vi "AlliGator Init Settings v2.vi"(8 "error in":errorcluster, 10 "Parameters to set to Default":T1[](array[typedef]), 11 "Settings Panel (Empty: All)":string) -> (0 "error out":errorcluster)   [LabVIEW 2021, in "AlliGator Settings.lvlib"]
doc: "Resets selected Settings parameters to their default values."
uses:
  AlliGator Settings.lvlib
  AlliGator Settings List.ctl
  Arrays/Linear Ramp End Options.ctl
  AlliGator Settings Event.ctl
  AlliGator Settings Window Messages.ctl
  AlliGator Define Gates to.ctl
  AlliGator Gates to Skip.ctl
  AlliGator Average Lifetime Options.ctl
  Fits/IRF(X)PSED/IRF(X)PSED Extraction Options.ctl
  Fits/IRF(X)PSED/Fourier Series Smoothing Option.ctl
  Fits/IRF(X)PSED/Fourier Series Truncation.ctl
  Fits/IRF(X)PSED/IRF Extraction Method.ctl
  AlliGator IRF Optimization Controls.ctl
  AlliGator IRF Deconvolution Metrics.ctl
  Fits/Square Pulse/Square Pulse Options.ctl
  Fits/Square Pulse/Square Pulse Levels Type.ctl
  Math/Advanced Signal Processing Toolkit/Wavelet Analysis Options.ctl
  AlliGator Baseline Subtraction Method.ctl
  Graphs/XY Graph/XY Graph Plot Shift Parameters.ctl
  Graphs/XY Graph/XY Graph Plot Shift Method.ctl
  Fits/IRF(X)PSED/Decay Fit Options v2.ctl
  Fits/Decay Convolution/Decay Model.ctl
  Fits/Residual Type.ctl
  Fits/IRF(X)PSED/Fit Weights Type.ctl
  Fits/Non-linear Fitting Method v2.ctl
  Fits/Fit Calculation Method.ctl
  Fits/Non-linear Fitting Algorithm.ctl
  Fits/IRF(X)PSED/Decay Fit Parameters & Derived Quantities List.ctl
  AlliGator Decay Fit Parameter Constraints 2.ctl
  Fits/IRF(X)PSED/Decay Fit Parameters In List.ctl
  AlliGator Guess Parameters Options.ctl
  Fits/IRF(X)PSED/MLE Baseline Offset Type.ctl
  AlliGator Exported Image Settings.ctl
  Histograms/Linear Histogram Options.ctl
  Histograms/Histogram Bin Option.ctl
  Histograms/Histogram Bin Position.ctl
  Image/Image Save File Format.ctl
  AlliGator Calibration Map Algorithm.ctl
  Phasor/Phasor Calibration Type.ctl
  AlliGator Phasor Reference Associated with Shortest Lifetime.ctl
  Phasor/Phasor Ratio Type.ctl
  Phasor/Phasor Standard Deviation Options.ctl
  AlliGator Phasor Plot Graphics Options.ctl
  AlliGator Phasor Plot Size.ctl
  AlliGator Phasor Plot Smoothing Options.ctl
  Arrays/Kernel Type.ctl
  Arrays/Smoothing Algorithm.ctl
  AlliGator Phasor Ratio Color-Coded Quantity.ctl
  AlliGator Python Settings.ctl
  Phasor/Phasor Explorer Decay Parameters.ctl
  Phasor/Phasor IRF Model.ctl
  Phasor/Phasor Explorer Display Parameters.ctl
  Phasor/Phasor Type of Series.ctl
  Phasor/Phasor Explorer Gate Parameters.ctl
  Phasor/Phasor Gate Type.ctl
  Phasor/Phasor Type of User-defined Function.ctl
  Phasor/Phasor Explorer Phasor Parameters.ctl
  Phasor/Phasor Calculation Type.ctl
  Phasor/Phasor SEPL Type.ctl
  Graphs/XY Graph/XY Plot Data.ctl
  AlliGator High Count Pixels Rejection Options.ctl
  SwissSPAD/SwissSPAD Live_Image Display Options.ctl
  AlliGator Image Binning Options.ctl
  AlliGator Image Smoothing Options.ctl
  AlliGator Low Count Pixels Rejection Options.ctl
  AlliGator Source Image Scale Bar Options.ctl
  Image/Flatfield Correction Options.ctl
  528bb3ad-a7d6-4b51-8aeb-33b87c87e59f.vi
  7656f502-c6d9-4b62-8342-3e3474e45c54.vi
  7a1d85e8-f51a-467b-92ae-4795812e884b.vi
  48533959-b6d0-4ae5-a5e9-0e715072b6cc.vi
  d87100d8-5b63-464b-a767-9d3b270a4e3f.vi
  7656f502-c6d9-4b62-8342-3e3474e45c54.vi/539bd7ec-d9e8-460f-a56d-a449b4a86a5e.vi
  7a1d85e8-f51a-467b-92ae-4795812e884b.vi/539bd7ec-d9e8-460f-a56d-a449b4a86a5e.vi
  48533959-b6d0-4ae5-a5e9-0e715072b6cc.vi/539bd7ec-d9e8-460f-a56d-a449b4a86a5e.vi
  d87100d8-5b63-464b-a767-9d3b270a4e3f.vi/539bd7ec-d9e8-460f-a56d-a449b4a86a5e.vi
  AlliGator Decay Analysis.lvlib
  Graphs/XY Graph/XY Graph Add-Ons.lvlib
  AlliGator Phasor Plot.lvlib
  Image/Image.lvlib
  AlliGator Decay Preprocessing.lvlib
  Fits/Fits.lvlib
  AlliGator Decay Fit.lvlib
  AlliGator IRF.lvlib
  Math/Math.lvlib
  Arrays/Arrays.lvlib
  Strings/Strings.lvlib
  AlliGator Source Image.lvlib
  Phasor/Phasor Explorer.lvlib
  Phasor/Phasor.lvlib
  AlliGator Phasor Ratio.lvlib
  Histograms/Histogram Window.lvlib
  AlliGator Phasor Calibration.lvlib
  SwissSPAD/SwissSPAD Live.lvlib
panel:
  # "see the AlliGator License on the block diagram (Ctrl+E or Window:Show Block Diagram)"
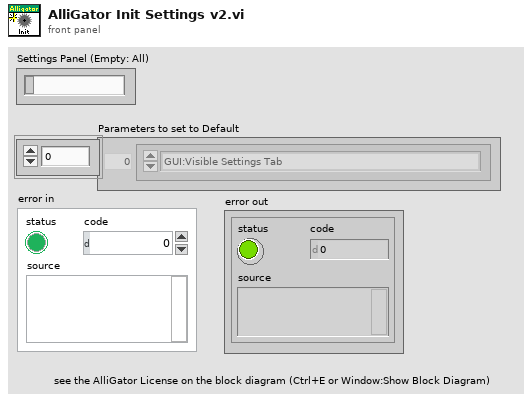
[diagram p1: front panel]
types:
  T1 = typedef "AlliGator Settings.lvlib/AlliGator Settings List.ctl" = enum16{"GUI:Visible Settings Tab", "GUI:Last Run Version", "Source Image:Use Image Histogram for Contrast", "Source Image:Low Count Pixels Rejection Options", "Source Image:High Count Pixels Rejection Options", "Source Image:Use Image Brightness", "Source Image:Blend Overlay with Image Background", "Source Image:Use Fixed ROI Diameter", "Source Image:ROI Diameter", "Source Image:ROI Center Color", "Source Image:Peak Threshold", "Source Image:Intensity Threshold", "Source Image:Image Binning Options", "Source Image:Image Smoothing Options", "Source Image:Image Histogram Active", "Source Image:Invert Binary Mask", "Source Image:Hot Pixel Removal", "Source Image:Overlay Analyzed ROI Center", "Source Image:Auto-Adjust Contrast", "Source Image:Histogram Lower Percentile", "Source Image:Histogram Upper Percentile", "Source Image:Save Source Image", "Source Image:Scale Bar Options", "Source Image:Image Resolution (Pixel Size)", "Source Image:Flatfield Correction", "Source Image:Show Dead Left Columns Correction", "Source Image:Dead Left Columns Correction", "Source Image:Image Pre-Processing Operations Order", "Source Image:Overlay ROI Median", "Source Image:Median Overlay Color", "Data Information:Gate Width", "Data Information:Nanotime Gate Separation", "Data Information:Macrotime Gate Separation", "Data Information:Gate Step", "Data Information:# Gates", "Data Information:Gate Image Exposure", "Data Information:Gate Image Integration", "Data Information:Gates to Skip", "Data Information:Gates to Keep", "Data Information:Define Gates to", "Data Information:Channel Name", "Data Information:Available Channel Names", "Data Information:Channel Arithmetic", "Data Information:Background File Subtraction", "Data Information:Background File", "Data Information:Background Scaling Factor", "Data Information:Background Pile-up Correction", "Data Information:Background Pixel Well Capacity", "Data Information:Laser Period", "Data Information:SYNC Period", "Data Information:Pile-up Correction", "Data Information:Pixel Well Capacity", "Data Information:Dataset Scaling Factor", "Fluorescence Decay_Decay Pre-Processing:Reverse Gates", "Fluorescence Decay_Decay Pre-Processing:Verbose Decay Pre-Processing", "Fluorescence Decay_Decay Pre-Processing:Use Decay Pre-Processing", "Fluorescence Decay_Decay Pre-Processing:Background Subtraction", "Fluorescence Decay_Decay Pre-Processing:Background Definition Range", "Fluorescence Decay_Decay Pre-Processing:Baseline Subtraction Method", "Fluorescence Decay_Decay Pre-Processing:Decay Pre-Processing Operations Order", "Fluorescence Decay_Decay Pre-Processing:Smoothing Parameter", "Fluorescence Decay_Decay Pre-Processing:Shift Decay", "Fluorescence Decay_Decay Pre-Processing:Decay Shift Parameters", "Fluorescence Decay_Decay Pre-Processing:Fold Decay", "Fluorescence Decay_Decay Pre-Processing:# Folds", "Fluorescence Decay_Decay Pre-Processing:1-Normalize Decay", "Fluorescence Decay_Decay Pre-Processing:[0-1]-Normalize Decay", "Fluorescence Decay_Decay Pre-Processing:Smoothen Decay", "Fluorescence Decay_Decay Pre-Processing:Extrapolate Decay", "Fluorescence Decay_Decay Pre-Processing:Use Periodicity", "Fluorescence Decay_Decay Pre-Processing:Use Cursors", "Fluorescence Decay_Decay Pre-Processing:Tail Fraction", "Fluorescence Decay_Decay Pre-Processing:Head Fraction", "Fluorescence Decay_Decay Pre-Processing:Additional Points", "Fluorescence Decay_Decay Pre-Processing:Straighten Decay", "Fluorescence Decay_Decay Pre-Processing:Constant Background", "Fluorescence Decay_Decay Pre-Processing:Pixel-Normalize Decay", "Fluorescence Decay_Advanced Analysis:Extract IRF instead of Decay", "Fluorescence Decay_Advanced Analysis:IRF Extraction Options", "Fluorescence Decay_Advanced Analysis:IRF Optimization Options", "Fluorescence Decay_Advanced Analysis:Square Pulse Options", "Fluorescence Decay_Advanced Analysis:IRF Order", "Fluorescence Decay_Advanced Analysis:IRF Time Constants", "Fluorescence Decay_Advanced Analysis:Wavelet Analysis Options", "Fluorescence Decay_Advanced Analysis:Average Lifetime Options", "Fluorescence Decay_Fit Options:Fit Options", "Fluorescence Decay_Fit Options:Use Legacy Fitting Approach", "Fluorescence Decay_Fit Options:Use Data Information Laser Period", "Fluorescence Decay_Fit Parameters:Displayed Fit Parameters", "Fluorescence Decay_Fit Parameters:Fit Parameter Constraints", "Fluorescence Decay_Fit Parameters:Export Tabulated Results", "Fluorescence Decay_Fit Parameters:MLE Baseline Offset Type", "Fluorescence Decay_Fit Parameters:MLE Baseline Offset", "Fluorescence Decay_Fit Parameters:Guess Parameter Names", "Fluorescence Decay_Fit Parameters:Guess Parameter Values", "Fluorescence Decay_Fit Parameters:Guess Parameters Options", "Fluorescence Decay_Styles:Show Last Decay Only", "Fluorescence Decay_Styles:Decay Graph Color Array", "Fluorescence Decay:Decay Graph Active", "Fluorescence Decay Statistics:Min Peak Value", "Fluorescence Decay Statistics:Reject Low Decay Peak Pixels", "Fluorescence Decay Statistics:Reject High Decay Peak Pixels", "Fluorescence Decay Statistics:Max Peak Value", "Time Traces:Use File Timestamp", "Time Traces:Time Step", "Time Traces:Use Intensity Correction File", "Time Traces:Intensity Correction File", "Phasor Plot:Phasor Plot Smoothing Options", "Phasor Plot:Phasor Plot Size", "Phasor Plot:Phasor Plot Graphics Options", "Phasor Plot:Cumulative Phasor Plot", "Phasor Plot:Use Phasor Brightness", "Phasor Plot:Blend Overlay with Phasor Background", "Phasor Plot:Save Phasor Plot", "Phasor Plot:Show References", "Phasor Plot:Phasor Ratio Decay Range", "Phasor Plot:Exponential Fading", "Phasor Plot:Phasor Ratio Reference Colors", "Phasor Plot:Reference Radius", "Phasor Plot:Show Color Map Vertices", "Phasor Plot:Phasor Plot Active", "Phasor Plot:Phasor Ratio Color Map Type", "Phasor Plot:Phasor Ratio Color Map", "Phasor Plot:Phasor Ratio Display Range", "Phasor Plot:Selected Image ROI(s)", "Phasor Plot:All Image ROIs", "Phasor Plot:Selected Phasor Plot ROI(s)", "Phasor Plot:All Phasor Plot ROIs", "Phasor Plot:Phasor Ratio Color-Coded Quantity", "Phasor Plot:Store Phasor Harmonics", "Phasor Plot:Draw Reference Segment", "Phasor Plot:User-Defined Quantity", "Phasor Graph:Phasor Frequency", "Phasor Graph:Phasor Ratio Type", "Phasor Graph:Pixel-level Phasor Computation", "Phasor Graph:Save Phasor Graph", "Phasor Graph:Phasor Graph Active", "Phasor Graph:Phasor SDV Options", "Phasor Calibration:Use Backup Calibration if needed", "Phasor Graph:Define Shortest Lifetime as", "Phasor Calibration:Backup Calibration Type", "Phasor Calibration:Calibration Type", "Phasor Calibration:Calibration Lifetime", "Phasor Calibration:Calibration Map Algorithm", "Single-Exponential Phasor Locus (SEPL):Gate Parameters", "Single-Exponential Phasor Locus (SEPL):User-defined Gate", "Single-Exponential Phasor Locus (SEPL):User-defined IRF", "Single-Exponential Phasor Locus (SEPL):Phasor Parameters", "Single-Exponential Phasor Locus (SEPL):Decay & IRF Parameters", "Single-Exponential Phasor Locus (SEPL):Display Parameters", "Lifetime Analysis:Decay Analysis Parameters", "Lifetime Analysis:Lifetime Map Active", "Plugins:Python Settings", "Miscellaneous:Verbose Mode", "Miscellaneous:Beep after Script", "Miscellaneous:Saved Image File Format", "Miscellaneous:Exported Gate Image Settings", "Miscellaneous:Include Loading in Timing", "Miscellaneous:Verbose Settings Mode", "Miscellaneous:Histogram Options", "Miscellaneous:Beep on Error", "Miscellaneous:# Logical Processors Used", "Miscellaneous:ROI Description Max Characters", "Miscellaneous:Verbose Error Mode", "Miscellaneous:Transparent Mask Color"}
  T2 = typedef "Arrays.lvlib/Linear Ramp End Options.ctl" = enum16{"Include Min/Exclude Max", "Exclude Min/Include Max", "Include Both Ends", "Exclude Both Ends"}
  T3 = typedef "AlliGator Settings.lvlib/AlliGator Settings Event.ctl" = cluster{"AlliGator Settings Message":T4, "Sender":string, "Control Label":string, "Data":variant}
  T4 = typedef "AlliGator Settings.lvlib/AlliGator Settings Window Messages.ctl" = enum16{"Idle", "Subscribe", "Unsubscribe", "Refresh Parameter", "Refresh All Parameters", "Quit"}
  T5 = typedef "AlliGator Settings.lvlib/AlliGator Define Gates to.ctl" = enum32{"Skip", "Keep"}
  T6 = typedef "AlliGator Decay Analysis.lvlib/AlliGator Gates to Skip.ctl" = cluster{"Start":u32, "End":u32}
  T7 = typedef "AlliGator Settings.lvlib/AlliGator Average Lifetime Options.ctl" = cluster{"Use Local IRF ":bool, "Use IRF Offset":bool, "Use Fixed Offset":bool, "Fixed Offset":dbl[unit], "Baseline %":dbl}
  T8 = typedef "Fits.lvlib/IRF(X)PSED Extraction Options.ctl" = cluster{"Time Constant for IRF Extraction":dbl[unit], "IRF Order":i32, "Fourier Series Smoothing":T9, "Noise Threshold":dbl, "Smoothing Width":dbl, "Fourier Series Truncation":T10, "Truncation Order":i32, "Save Power Spectrum":bool, "Smoothing":bool, "Smoothing Parameter":dbl, "Smoothing Order":u32, "Method":T11}
  T9 = typedef "Fits.lvlib/Fourier Series Smoothing Option.ctl" = enum16{"None", "Lanczos Factors", "Fejer Summation"}
  T10 = typedef "Fits.lvlib/Fourier Series Truncation.ctl" = enum16{"Automatic", "Fixed"}
  T11 = typedef "Fits.lvlib/IRF Extraction Method.ctl" = enum16{"Direct", "Topless", "Toeplitz"}
  T12 = typedef "AlliGator Decay Analysis.lvlib/AlliGator IRF.lvlib/AlliGator IRF Optimization Controls.ctl" = cluster{"Search Range":dbl[unit], "Search Step":dbl[unit], "Tail Threshold (%)":dbl, "Regularized IRF":bool, "Export Plot":bool, "Export Data":bool, "Smooth Metrics":bool, "S-G Side Points":i32, "S-G Polynomial Order":i32, "Metrics":T13}
  T13 = typedef "AlliGator Decay Analysis.lvlib/AlliGator IRF.lvlib/AlliGator IRF Deconvolution Metrics.ctl" = enum16{"Average", "SDV", "Max", "Average * SDV", "Slope"}
  T14 = typedef "Fits.lvlib/Square Pulse Options.ctl" = cluster{"Method":T15, "# Bins":i32, "Threshold %":dbl, "Center on Midpoint":bool, "Smoothen Plot":bool}
  T15 = typedef "Fits.lvlib/Square Pulse Levels Type.ctl" = enum16{"Mode", "Mean"}
  T16 = typedef "Math.lvlib/Wavelet Analysis Options.ctl" = cluster{"Wavelet":enum16{"db02", "db03", "db04", "db05", "db06", "db07", "db08", "db09", "db10", "db11", "db12", "db13", "db14", "Haar", "bior1_3", "bior1_5", "bior2_2", "bior2_4", "bior2_6", "bior2_8", "bior3_1", "bior3_3", "bior3_5", "bior3_7", "bior3_9", "bior4_4 (FBI)", "bior5_5", "bior6_8", "coif1", "coif2", "coif3", "coif4", "coif5", "sym2", "sym3", "sym4", "sym5", "sym6", "sym7", "sym8"}, "Option for Approximate Coefficients":enum16{"None", "Threshold", "Detrend"}, "# Levels":i32, "Threshold Settings":cluster{"Thresholding Rule":enum16{"SURE", "Hybrid", "Universal", "Minimax"}, "Rescaling Method":enum16{"One", "Single level", "Multiple levels"}, "Soft Threshold?":bool}, "Wavelet Transform Type":enum16{"Discrete", "Undecimated"}}
  T17 = cluster{"Min Gate":dbl[unit], "Max Gate":dbl[unit]}
  T18 = typedef "AlliGator Decay Analysis.lvlib/AlliGator Decay Preprocessing.lvlib/AlliGator Baseline Subtraction Method.ctl" = enum16{"Mean", "Min", "Square Gated Single-Exponential", "File", "Constant"}
  T19 = typedef "XY Graph Add-Ons.lvlib/XY Graph Plot Shift Parameters.ctl" = cluster{"Type":T20, "Shift":dbl[unit], "Threshold":dbl, "Rotate":bool}
  T20 = typedef "XY Graph Add-Ons.lvlib/XY Graph Plot Shift Method.ctl" = enum16{"Default", "CFD", "Threshold", "Cross-Correlation"}
  T21 = typedef "Fits.lvlib/Decay Fit Options v2.ctl" = cluster{"Show Fit Residuals":bool, "Fit Model":T22, "Residual Type":T23, "Max Decay Percentile":dbl, "Min Decay Percentile":dbl, "Show Full Decay":bool, "Weights":T24, "Fitting Method":T25, "Compute Parameter Uncertainties":bool, "Periodic Boundaries":bool, "Model Calculation":T26, "Period":dbl[unit], "Termination Criteria":cluster{"Max Iterations":i32, "Max Function Calls":i32, "Max Time":dbl[unit], "Function Tolerance":dbl, "Parameter Tolerance":dbl, "Gradient Tolerance":dbl, "Min Lambda":dbl, "Max Lambda":dbl, "Initial Tick Count":u32}, "Offset Resolution":dbl[unit], "Use Local IRF":bool, "Fitting Algorithm":T27}
  T22 = typedef "Fits.lvlib/Decay Model.ctl" = enum16{"1-Exponential", "2-Exponentials"}
  T23 = typedef "Fits.lvlib/Residual Type.ctl" = enum16{"Standard", "Normalized", "Reduced"}
  T24 = typedef "Fits.lvlib/Fit Weights Type.ctl" = enum16{"Unweighted", "1/Variance", "Best of All"}
  T25 = typedef "Fits.lvlib/Non-linear Fitting Method v2.ctl" = enum16{"Least Square", "Least Absolute Residual", "Bisquare", "MLE", "-", "Best of All"}
  T26 = typedef "Fits.lvlib/Fit Calculation Method.ctl" = enum16{"Simulation", "Convolution", "Integration"}
  T27 = typedef "Fits.lvlib/Non-linear Fitting Algorithm.ctl" = enum16{"Levenberg-Marquardt", "Trust-Region Dogleg"}
  T28 = typedef "AlliGator Decay Analysis.lvlib/AlliGator Decay Fit.lvlib/AlliGator Decay Fit Parameter Constraints 2.ctl" = cluster{"Fit Parameter":T29, "Min Value":dbl, "Max Value":dbl, "Global":bool, "Used":bool}
  T29 = typedef "Fits.lvlib/Decay Fit Parameters In List.ctl" = enum16{"Offset", "Baseline", "A_1", "tau_1", "A_2", "tau_2"}
  T30 = typedef "AlliGator Decay Analysis.lvlib/AlliGator Decay Fit.lvlib/AlliGator Guess Parameters Options.ctl" = enum16{"Numerically estimated", "User-provided", "User-provided (normalized)", "Last valid fitted parameters"}
  T31 = typedef "Fits.lvlib/MLE Baseline Offset Type.ctl" = enum32{"Absolute", "Percentage"}
  T32 = typedef "AlliGator Settings.lvlib/AlliGator Exported Image Settings.ctl" = cluster{"bitness":bool, " Min Value":sgl, " Max Value":sgl}
  T33 = typedef "Histogram Window.lvlib/Linear Histogram Options.ctl" = cluster{"Bin Size":dbl, "Bin Number":i32, "Bin Option":T34, "Min Value":dbl, "Max Value":dbl, "Filter NaN & Infinite Values":bool, "Frequency Plot":bool, "Align Bins":bool, "Bin Location":T35, "Project Outside Values":bool, "Max Histogram Size":i32}
  T34 = typedef "Histogram Window.lvlib/Histogram Bin Option.ctl" = enum32{"Bin Number", "Bin Size"}
  T35 = typedef "Histogram Window.lvlib/Histogram Bin Position.ctl" = enum16{"Left", "Center", "Right"}
  T36 = typedef "Image.lvlib/Image Save File Format.ctl" = enum16{"PNG", "JPEG", "BMP"}
  T37 = enum16{"Single Calibration", "Nearest Valid Calibration"}
  T38 = typedef "AlliGator Phasor Calibration.lvlib/AlliGator Calibration Map Algorithm.ctl" = enum16{"Simple Search", "Min Distance"}
  T39 = typedef "Phasor.lvlib/Phasor Calibration Type.ctl" = enum16{"None", "Single Phasor", "Phasor Series", "Phasor Map"}
  T40 = typedef "AlliGator Phasor Ratio.lvlib/AlliGator Phasor Reference Associated with Shortest Lifetime.ctl" = enum32{"Reference 1", "Reference 2"}
  T41 = typedef "Phasor.lvlib/Phasor Ratio Type.ctl" = enum32{"Intensity-weighted", "Amplitude-weighted"}
  T42 = typedef "Phasor.lvlib/Phasor Standard Deviation Options.ctl" = cluster{"Compute Estimated SDV":bool, "# Replicas":u32, "Use Estimated Average Phasor":bool}
  T43 = typedef "AlliGator Settings.lvlib/AlliGator Phasor Plot Graphics Options.ctl" = cluster{"UC Color":u32, "Show UC Tau Ticks":bool, "SEPL Color":u32, "Show SEPL Tau Ticks":bool, "Axes Color":u32, "Show (g,s) Ticks":bool, "Show UC":bool, "Show SEPL":bool, "Show Axes":bool, "Show UC Tau Labels":bool, "Show SEPL Tau Labels":bool, "Show (g,s) Labels":bool, "UC Label Size":i16, "UC Label Distance":dbl, "SEPL Label Size":i16, "SEPL Label Distance":dbl, "Axes Label Size":i16, "Axes Label Distance":dbl}
  T44 = typedef "AlliGator Phasor Plot.lvlib/AlliGator Phasor Plot Size.ctl" = cluster{"H":i32, "V":i32, "Margin":dbl}
  T45 = typedef "AlliGator Phasor Plot.lvlib/AlliGator Phasor Plot Smoothing Options.ctl" = cluster{"Use Phasor Plot Smoothing":bool, "Kernel Type":T46, "Bin":i32, "Algorithm":T47}
  T46 = typedef "Arrays.lvlib/Kernel Type.ctl" = enum16{"Uniform", "Bilinear", "Gaussian"}
  T47 = typedef "Arrays.lvlib/Smoothing Algorithm.ctl" = enum16{"Rapid", "Thorough"}
  T48 = enum32{"Interpolate Reference Colors", "Use Custom Map"}
  T49 = typedef "AlliGator Phasor Ratio.lvlib/AlliGator Phasor Ratio Color-Coded Quantity.ctl" = enum16{"Phasor Ratio (f1 or a1)", "Average Lifetime (<tau>_i or <tau>_a))", "User-Defined Quantity"}
  T50 = cluster{"Reference 1":u32, "Reference 2":u32, "Boundary":u32}
  T51 = typedef "AlliGator Settings.lvlib/AlliGator Python Settings.ctl" = cluster{"Python Version":string, "Use PATH definition":bool, "Python.exe Path":path, "Include Example Plugins":bool}
  T52 = typedef "Phasor Explorer.lvlib/Phasor Explorer Decay Parameters.ctl" = cluster{"Lifetime":dbl[unit], "IRF Offset":dbl[unit], "IRF Period":dbl[unit], "Normalized Decays":bool, "IRF Model":T53, "IRF Parameter 1":dbl[unit]}
  T53 = typedef "Phasor.lvlib/Phasor IRF Model.ctl" = enum16{"Dirac", "Exponential"}
  T54 = typedef "Phasor Explorer.lvlib/Phasor Explorer Display Parameters.ctl" = cluster{"# Points":i32, "Ramp Type":enum16{"Linear", "Logarithmic"}, "Type of Series":T55, "Min tau":dbl[unit], "Max tau":dbl[unit], "Include 0":bool, "Include Infinity":bool}
  T55 = typedef "Phasor.lvlib/Phasor Type of Series.ctl" = enum16{"1-Exp Decays", "Linear Combination of 1-Exp"}
  T56 = typedef "Phasor Explorer.lvlib/Phasor Explorer Gate Parameters.ctl" = cluster{"First Gate Start":dbl[unit], "Use Gate Center":bool, "Gate Width":dbl[unit], "Gate Step":dbl[unit], "# Gates":dbl, "Gate Type":T57, "Edge Width":dbl[unit], "Top Slope":dbl[unit], "Reversed Sawtooth?":bool, "Analytical Computation":bool, "Integration":enum32{"Item 0", "Item 1"}, "Tolerance":dbl, "# Steps":dbl, "Type of User-defined Function":T58, "Use Gate Step":bool}
  T57 = typedef "Phasor.lvlib/Phasor Gate Type.ctl" = enum16{"Square", "Finite Edge Square", "Finite Edge, Tilted Top Square", "Triangle", "Sawtooth", "User-defined"}
  T58 = typedef "Phasor.lvlib/Phasor Type of User-defined Function.ctl" = enum16{"Gate", "IRF"}
  T59 = typedef "Phasor Explorer.lvlib/Phasor Explorer Phasor Parameters.ctl" = cluster{"Harmonic Frequency":dbl[unit], "Use f* = 1/D Frequency":bool, "Calibrated Phasor":bool, "Calibration Lifetime":dbl[unit], "Phasor Calculation":T60, "SEPL Type":T61, "# Gates":dbl, "Square Gate Width":dbl[unit], "Show Ticks":bool}
  T60 = typedef "Phasor.lvlib/Phasor Calculation Type.ctl" = enum16{"Direct Sum", "Analytical Formula"}
  T61 = typedef "Phasor.lvlib/Phasor SEPL Type.ctl" = enum16{"UC", "L_N", "L_N[W]", "L_X"}
  T62 = typedef "XY Graph Add-Ons.lvlib/XY Plot Data.ctl" = cluster{"X Array":dbl[], "Y Array":dbl[]}
  T63 = typedef "AlliGator Settings.lvlib/AlliGator High Count Pixels Rejection Options.ctl" = cluster{"Background High Threshold Factor":dbl, "Fixed High Background Threshold":dbl, "Reject High Count Pixels":bool, "High Percentile":dbl}
  T64 = typedef "SwissSPAD Live.lvlib/SwissSPAD Live_Image Display Options.ctl" = cluster{"Remove Screamers":bool, "Delta":sgl, "Equalize Histogram":bool, "Percentile":sgl, "Hot Pixel Mask Image":path, "Use Hot Pixel Mask":bool}
  T65 = typedef "AlliGator Source Image.lvlib/AlliGator Image Binning Options.ctl" = cluster{"Use Image Binning":bool, "X Bin":i32, "Y Bin":i32}
  T66 = typedef "AlliGator Settings.lvlib/AlliGator Image Smoothing Options.ctl" = cluster{"Use Image Smoothing":bool, "Kernel Type":T46, "Bin":i32, "Algorithm":T47}
  T67 = typedef "AlliGator Settings.lvlib/AlliGator Low Count Pixels Rejection Options.ctl" = cluster{"Background Low Threshold Factor":dbl, "Fixed Low Background Threshold":dbl, "Reject Low Count Pixels":bool, "Low Percentile":dbl}
  T68 = typedef "AlliGator Source Image.lvlib/AlliGator Source Image Scale Bar Options.ctl" = cluster{"Show Scale Bar Overlay":bool, "Scale Bar Length":dbl[unit], "Scale Bar Color":u32, "Scale Bar X":u32, "Scale Bar Y":u32, "Scale Bar Height":dbl[unit]}
  T69 = typedef "Image.lvlib/Flatfield Correction Options.ctl" = cluster{"Flatfield Estimation Options":cluster{"Sampling Grid Size X":i32, "Sampling Grid Size Y":i32, "Polynomial Degree":i32}, "Background Options":cluster{"Estimate Background":bool, "Background Estimation Size":i32, "Niblack Deviation Factor [0. 1]":dbl}, "Correction Factor":sgl}
  T70 = typedef "Fits.lvlib/Decay Fit Parameters & Derived Quantities List.ctl" = enum16{"Offset", "Baseline", "A_1", "tau_1", "A_2", "tau_2", "<tau>_a", "f1_a", "f2_a", "<tau>_i", "f1_i", "f2_i", "-", "R^2", "Chi^2"}
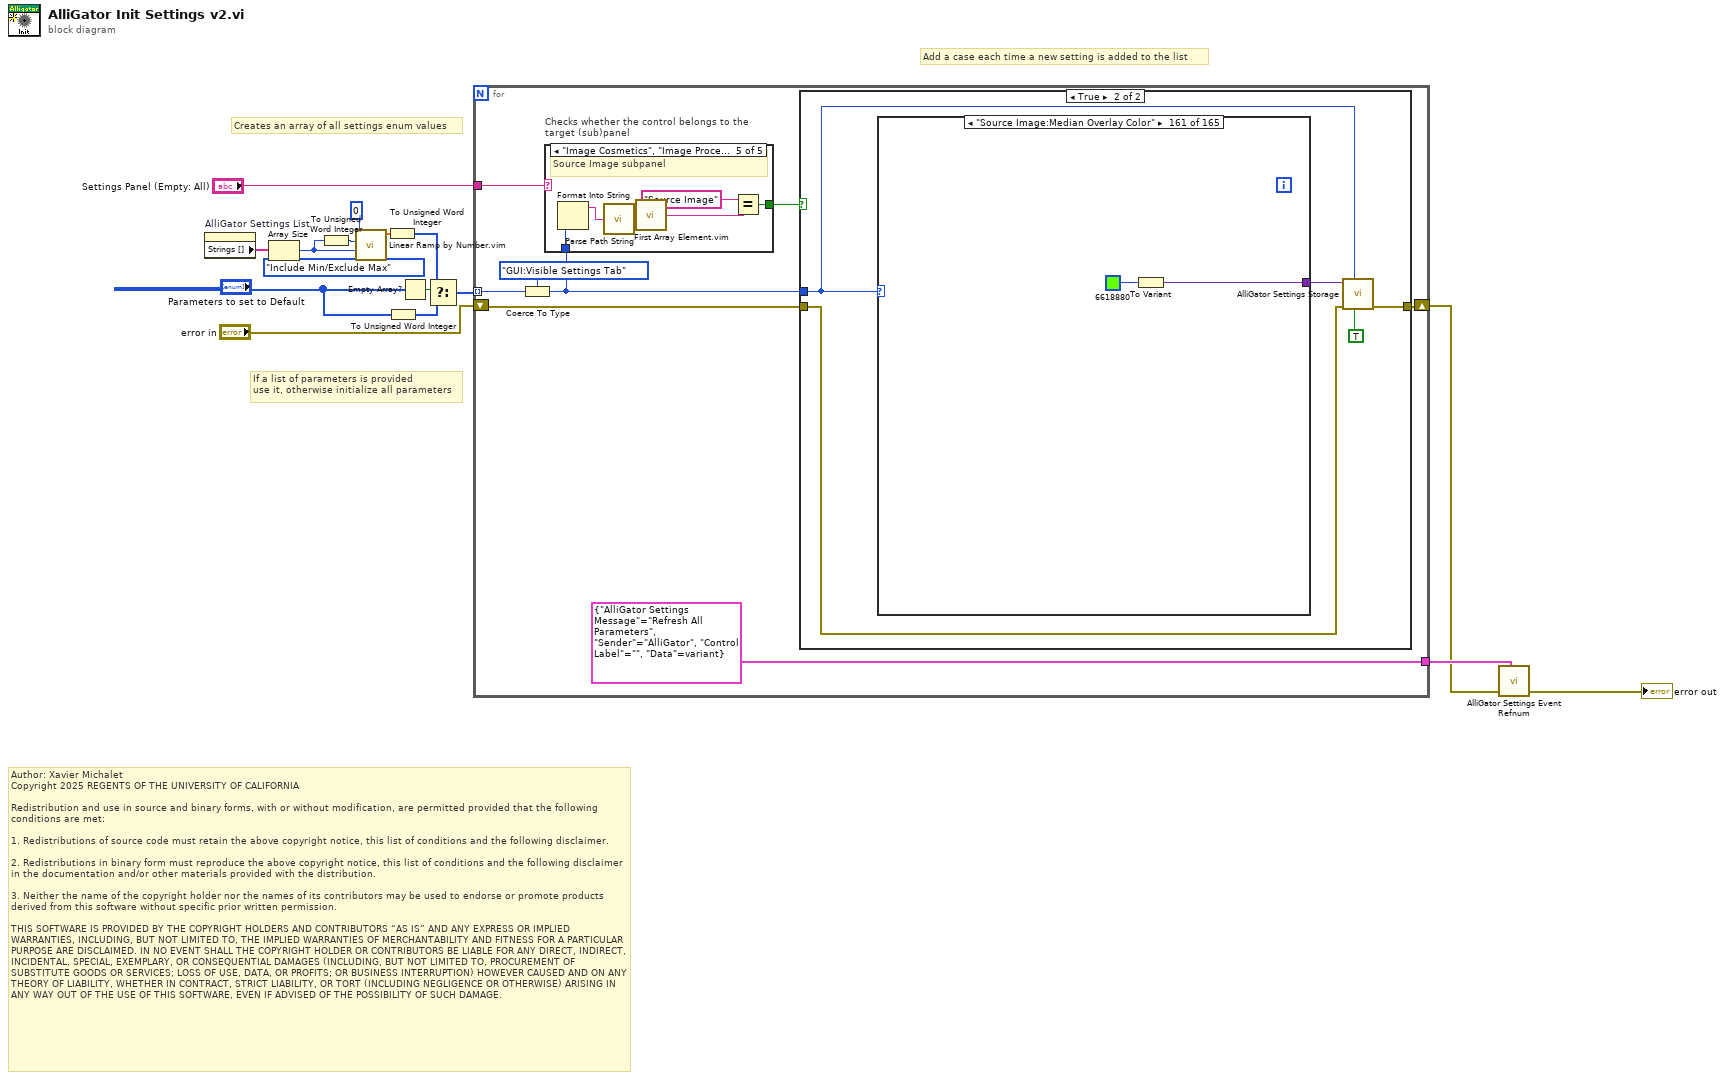
[diagram p0: block diagram]
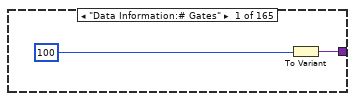
[diagram p3: hidden frame]
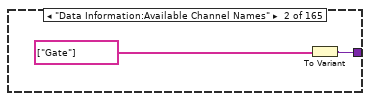
[diagram p4: hidden frame]
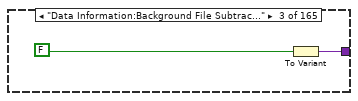
[diagram p5: hidden frame]
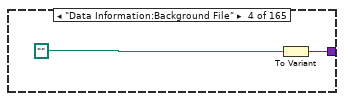
[diagram p6: hidden frame]
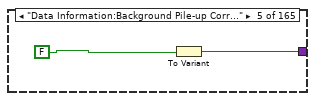
[diagram p7: hidden frame]
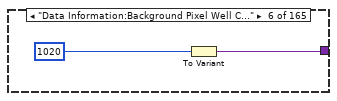
[diagram p8: hidden frame]
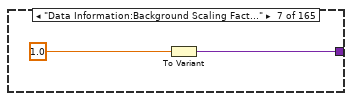
[diagram p9: hidden frame]
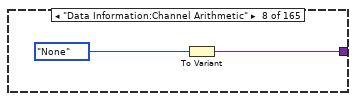
[diagram p10: hidden frame]
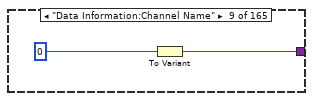
[diagram p11: hidden frame]
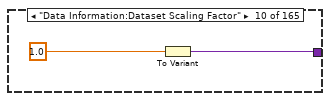
[diagram p12: hidden frame]
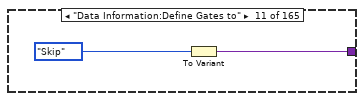
[diagram p13: hidden frame]
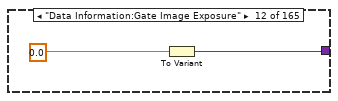
[diagram p14: hidden frame]
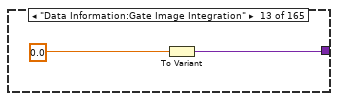
[diagram p15: hidden frame]
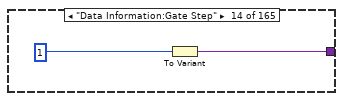
[diagram p16: hidden frame]
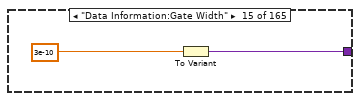
[diagram p17: hidden frame]
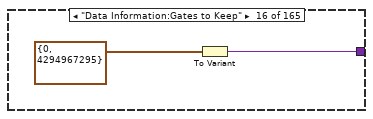
[diagram p18: hidden frame]
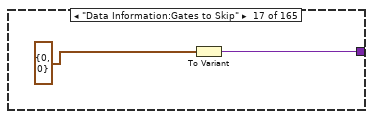
[diagram p19: hidden frame]
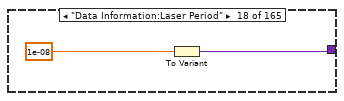
[diagram p20: hidden frame]
diagram:
  # "Creates an array of all settings enum values"
  # "Author: Xavier Michalet\nCopyright 2025 REGENTS OF THE UNIVERSITY OF CALIFORNIA\n\nRedistribution and use in source and binary forms, with or without modification, are permitted provided that the following conditions are met:\n\n1. Redistributions of source code must retain the above copyright notice, this list of conditions and the following disclaimer.\n\n2. Redistributions in binary form must reproduce the above copyright notice, this list of conditions and the following disclaimer in the documentation and/or other materials provided with the distribution.\n\n3. Neither the name of the copyright holder nor the names of its contributors may be used to endorse or promote products derived from this software without specific prior written permission.\n\nTHIS SOFTWARE IS PROVIDED BY THE COPYRIGHT HOLDERS AND CONTRIBUTORS “AS IS” AND ANY EXPRESS OR IMPLIED WARRANTIES, INCLUDING, BUT NOT LIMITED TO, THE IMPLIED WARRANTIES OF MERCHANTABILITY AND FITNESS FOR A PARTICULAR PURPOSE ARE DISCLAIMED. IN NO EVENT SHALL THE COPYRIGHT HOLDER OR CONTRIBUTORS BE LIABLE FOR ANY DIRECT, INDIRECT, INCIDENTAL, SPECIAL, EXEMPLARY, OR CONSEQUENTIAL DAMAGES (INCLUDING, BUT NOT LIMITED TO, PROCUREMENT OF SUBSTITUTE GOODS OR SERVICES; LOSS OF USE, DATA, OR PROFITS; OR BUSINESS INTERRUPTION) HOWEVER CAUSED AND ON ANY THEORY OF LIABILITY, WHETHER IN CONTRACT, STRICT LIABILITY, OR TORT (INCLUDING NEGLIGENCE OR OTHERWISE) ARISING IN ANY WAY OUT OF THE USE OF THIS SOFTWARE, EVEN IF ADVISED OF THE POSSIBILITY OF SUCH DAMAGE."
  # "If a list of parameters is provided\nuse it, otherwise initialize all parameters"
  # "Add a case each time a new setting is added to the list"
  n1 = property on="AlliGator Settings List" class="Enum (strict)"() -> ("Strings []"=w12:string[])  [unwired: 2 in, 2 out]
  n2 = Array Size(array=w12) -> (size(s)=w7:i32)
  n3 = To Unsigned Word Integer(number=w7) -> (unsigned 16bit integer=w9:u16)
  n4 = call "Linear Ramp by Number.vim"("Options"=Linear_Ramp_End_Options."Include Min/Exclude Max", "# Steps (1)"=w7, "End (1)"=w9, "Start (0)"=u16 0) -> ("Ramp"=w10:dbl[])  [unwired: 5 in, 2 out]
  n5 = To Unsigned Word Integer(number=w10) -> (unsigned 16bit integer=w6:u16[])
  n6 = To Unsigned Word Integer(number="Parameters to set to Default") -> (unsigned 16bit integer=w4:u16[])
  n7 = Empty Array?(array="Parameters to set to Default") -> (empty?=w13:bool)
  n8 = Select(t=w6, s=w13, f=w4) -> (s? t:f=w5:u16[])
  n9 = for {
    tunnel: "Settings Panel (Empty: All)" -> [w24]
    tunnel: w5 -> [w21] mode=indexing
    tunnel: [T3 {"AlliGator Settings Message"=enum."Refresh All Parameters", "Sender"="AlliGator", "Control Label"="", "Data"=variant} ("AlliGator Settings Event")] -> w3
    shift-right: [w18] -> w1
    shift-left: "error in" -> [w17]
    n10 = Coerce To Type(0:w21, 1:AlliGator_Settings_List."GUI:Visible Settings Tab" ("AlliGator Settings List")) -> (2:w23:T1)
    n11 = case "Checks whether the control belongs to the target (sub)panel" shown="\"Image Cosmetics\", \"Image Processing\", \"Pixel Processing\"" w24 {
      selector: w24 -> [_ w365 w371 w379 _]
      tunnel: w23 -> [_ w369 w377 w385 w391]
      tunnel: [TRUE w364 w374 w382 w388] -> w22
      frame "", "All" {
      }
      frame "Miscellaneous", Default {
        n12 = Format Into String(w369) -> (resulting string=w368:string)  [unwired: 3 in, 1 out]
        n13 = call "Parse Path String.vi"("Path in"=w368) -> ("Folder Hierarchy"=w367:string[])  [unwired: 4 in, 1 out]
        n14 = call "First Array Element.vim"("Array"=w367) -> ("First Element"=w366:string)  [unwired: 8 in]
        n15 = Equal?(x=w366, y=w365) -> (x = y?=w364:bool)
      }
      frame "Fluorescence Decay" {
        # "strip the subpanel names"
        n16 = Format Into String(w377) -> (resulting string=w376:string)  [unwired: 3 in, 1 out]
        n17 = call "Parse Path String.vi"("Path in"=w376) -> ("Folder Hierarchy"=w375:string[])  [unwired: 4 in, 1 out]
        n18 = call "First Array Element.vim"("Array"=w375) -> ("First Element"=w373:string)  [unwired: 8 in]
        n19 = call "Split String Around Character.vi"("search string/char ( _ )"="_", "String in"=w373) -> ("String before"=w370:string)  [unwired: 8 in, 1 out]
        n20 = Equal?(x=w371, y=w370) -> (x = y?=w374:bool)
      }
      frame "Advanced Analysis", "Decay Pre-Processing", "Fit Options", "Fit Parameters", "Styles" {
        # "Fluorescence Decay subpanel"
        n21 = Format Into String(w385) -> (resulting string=w384:string)  [unwired: 3 in, 1 out]
        n22 = call "Parse Path String.vi"("Path in"=w384) -> ("Folder Hierarchy"=w383:string[])  [unwired: 4 in, 1 out]
        n23 = call "First Array Element.vim"("Array"=w383) -> ("First Element"=w381:string)  [unwired: 8 in]
        n24 = call "Split String Around Character.vi"("search string/char ( _ )"="_", "String in"=w381) -> ("String after"=w378:string)  [unwired: 8 in, 1 out]
        n25 = Equal?(x=w379, y=w378) -> (x = y?=w382:bool)
      }
      frame "Image Cosmetics", "Image Processing", "Pixel Processing" {
        # "Source Image subpanel"
        n26 = Format Into String(w391) -> (resulting string=w390:string)  [unwired: 3 in, 1 out]
        n27 = call "Parse Path String.vi"("Path in"=w390) -> ("Folder Hierarchy"=w389:string[])  [unwired: 4 in, 1 out]
        n28 = call "First Array Element.vim"("Array"=w389) -> ("First Element"=w387:string)  [unwired: 8 in]
        n29 = Equal?(x="Source Image", y=w387) -> (x = y?=w388:bool)
      }
    }
    n30 = case shown="True" w22 {
      tunnel: w23 -> [_ w26]
      tunnel: [w25 w30] -> w18
      tunnel: w17 -> [w25 w27]
      frame False {
      }
      frame True {
        n31 = case shown="\"Source Image:Median Overlay Color\"" w26 {
          tunnel: [w31 w33 w35 w37 w39 w41 w43 w45 w47 w49 w51 w53 w55 w57 w59 w61 w63 w65 w67 w69 w71 w73 w75 w77 w79 w81 w83 w85 w87 w89 w91 w93 w95 w97 w99 w101 w103 w105 w107 w109 w111 w113 w115 w117 w119 w121 w123 w125 w127 w129 w131 w133 w135 w137 w139 w141 w143 w145 w147 w149 w151 w153 w155 w157 w159 w161 w163 w165 w167 w169 w171 w173 w175 w177 w179 w181 w183 w185 w189 w191 w193 w195 w197 w199 w201 w203 w205 w207 w209 w211 w213 w215 w217 w219 w221 w223 w225 w227 w229 w231 w233 w235 w237 w239 w241 w243 w245 w247 w249 w251 w253 w255 w257 w259 w261 w263 w265 w267 w269 w271 w273 w275 w277 w279 w281 w283 w285 w287 w289 w291 w293 w295 w297 w299 w301 w303 w305 w307 w309 w311 w313 w315 w317 w319 w321 w323 w325 w327 w329 w331 w333 w335 w337 w339 w341 w343 w346 w348 w350 w352 w354 w355 w357 w359 w361] -> w29
          frame "Data Information:# Gates" {
            n32 = To Variant(anything=100 ("Gate Duration")) -> (Variant=w31:variant)
          }
          frame "Data Information:Available Channel Names" {
            n33 = To Variant(anything=string[] ["Gate"]) -> (Variant=w33:variant)
          }
          frame "Data Information:Background File Subtraction" {
            n34 = To Variant(anything=FALSE) -> (Variant=w35:variant)
          }
          frame "Data Information:Background File" {
            n35 = To Variant(anything=path "") -> (Variant=w37:variant)
          }
          frame "Data Information:Background Pile-up Correction" {
            n36 = To Variant(anything=FALSE) -> (Variant=w39:variant)
          }
          frame "Data Information:Background Pixel Well Capacity" {
            n37 = To Variant(anything=u32 1020) -> (Variant=w41:variant)
          }
          frame "Data Information:Background Scaling Factor" {
            n38 = To Variant(anything=1.0) -> (Variant=w43:variant)
          }
          frame "Data Information:Channel Arithmetic" {
            n39 = To Variant(anything=enum16{"None", "INT - G2", "<INT> + INT - 2 G2"}."None" ("Gate Arithmetic")) -> (Variant=w45:variant)
          }
          frame "Data Information:Channel Name" {
            n40 = To Variant(anything=u16 0) -> (Variant=w47:variant)
          }
          frame "Data Information:Dataset Scaling Factor" {
            n41 = To Variant(anything=1.0) -> (Variant=w49:variant)
          }
          frame "Data Information:Define Gates to" {
            n42 = To Variant(anything=AlliGator_Define_Gates_to."Skip" ("Define Gates to")) -> (Variant=w51:variant)
          }
          frame "Data Information:Gate Image Exposure" {
            n43 = To Variant(anything=dbl[unit] 0.0 ("Max Lifetime")) -> (Variant=w53:variant)
          }
          frame "Data Information:Gate Image Integration" {
            n44 = To Variant(anything=dbl[unit] 0.0 ("Max Lifetime")) -> (Variant=w55:variant)
          }
          frame "Data Information:Gate Step" {
            n45 = To Variant(anything=1 ("Gate Duration")) -> (Variant=w57:variant)
          }
          frame "Data Information:Gate Width" {
            n46 = To Variant(anything=dbl[unit] 3e-10 ("Gate Duration")) -> (Variant=w59:variant)
          }
          frame "Data Information:Gates to Keep" {
            n47 = To Variant(anything=T6 {"Start"=0, "End"=4294967295} ("Decay Points to Skip")) -> (Variant=w61:variant)
          }
          frame "Data Information:Gates to Skip" {
            n48 = To Variant(anything=T6 {"Start"=0, "End"=0} ("Decay Points to Skip")) -> (Variant=w63:variant)
          }
          frame "Data Information:Laser Period" {
            n49 = To Variant(anything=dbl[unit] 1e-08 ("Max Lifetime")) -> (Variant=w65:variant)
          }
          frame "Data Information:Macrotime Gate Separation" {
            n50 = To Variant(anything=dbl[unit] 0.0 ("Max Lifetime")) -> (Variant=w67:variant)
          }
          frame "Data Information:Nanotime Gate Separation" {
            n51 = To Variant(anything=dbl[unit] 4e-11 ("Gate Duration")) -> (Variant=w69:variant)
          }
          frame "Data Information:Pile-up Correction" {
            n52 = To Variant(anything=FALSE) -> (Variant=w71:variant)
          }
          frame "Data Information:Pixel Well Capacity" {
            n53 = To Variant(anything=1020) -> (Variant=w73:variant)
          }
          frame "Data Information:SYNC Period" {
            n54 = To Variant(anything=dbl[unit] 1e-08 ("Max Lifetime")) -> (Variant=w75:variant)
          }
          frame "Fluorescence Decay Statistics:Max Peak Value" {
            n55 = To Variant(anything=inf ("Min Peak Value")) -> (Variant=w77:variant)
          }
          frame "Fluorescence Decay Statistics:Min Peak Value" {
            n56 = To Variant(anything=500.0 ("Min Peak Value")) -> (Variant=w79:variant)
          }
          frame "Fluorescence Decay Statistics:Reject High Decay Peak Pixels" {
            n57 = To Variant(anything=FALSE) -> (Variant=w81:variant)
          }
          frame "Fluorescence Decay Statistics:Reject Low Decay Peak Pixels" {
            n58 = To Variant(anything=FALSE) -> (Variant=w83:variant)
          }
          frame "Fluorescence Decay:Decay Graph Active" {
            n59 = To Variant(anything=TRUE) -> (Variant=w85:variant)
          }
          frame "Fluorescence Decay_Advanced Analysis:Average Lifetime Options" {
            n60 = To Variant(anything=T7 {"Use Local IRF "=TRUE, "Use IRF Offset"=TRUE, "Use Fixed Offset"=FALSE, "Fixed Offset"=0.0, "Baseline %"=50.0} ("Average Lifetime Options")) -> (Variant=w87:variant)
          }
          frame "Fluorescence Decay_Advanced Analysis:Extract IRF instead of Decay" {
            n61 = To Variant(anything=FALSE) -> (Variant=w89:variant)
          }
          frame "Fluorescence Decay_Advanced Analysis:IRF Extraction Options" {
            n62 = To Variant(anything=T8 {"Time Constant for IRF Extraction"=1e-09, "IRF Order"=132, "Fourier Series Smoothing"=enum."None", "Noise Threshold"=0.1, "Smoothing Width"=1.0, "Fourier Series Truncation"=enum."Automatic", "Truncation Order"=0, "Save Power Spectrum"=FALSE, "Smoothing"=TRUE, "Smoothing Parameter"=-1.0, "Smoothing Order"=10, "Method"=enum."Direct"} ("IRF Extraction Options")) -> (Variant=w91:variant)
          }
          frame "Fluorescence Decay_Advanced Analysis:IRF Optimization Options" {
            n63 = To Variant(anything=T12 {"Search Range"=5e-10, "Search Step"=1e-12, "Tail Threshold (%)"=5.0, "Regularized IRF"=TRUE, "Export Plot"=TRUE, "Export Data"=FALSE, "Smooth Metrics"=TRUE, "S-G Side Points"=6, "S-G Polynomial Order"=3, "Metrics"=enum."SDV"} ("IRF Optimization Control")) -> (Variant=w93:variant)
          }
          frame "Fluorescence Decay_Advanced Analysis:IRF Order" {
            n64 = To Variant(anything=1 ("Time Constant for IRF Extraction")) -> (Variant=w95:variant)
          }
          frame "Fluorescence Decay_Advanced Analysis:IRF Time Constants" {
            n65 = To Variant(anything=dbl[] []) -> (Variant=w97:variant)
          }
          frame "Fluorescence Decay_Advanced Analysis:Square Pulse Options" {
            n66 = To Variant(anything=T14 {"Method"=enum."Mode", "# Bins"=100, "Threshold %"=10.0, "Center on Midpoint"=TRUE, "Smoothen Plot"=FALSE} ("Square Pulse Options")) -> (Variant=w99:variant)
          }
          frame "Fluorescence Decay_Advanced Analysis:Wavelet Analysis Options" {
            n67 = To Variant(anything=T16 {"Wavelet"=enum."db02", "Option for Approximate Coefficients"=enum."Threshold", "# Levels"=-1, "Threshold Settings"={"Thresholding Rule"=enum."Universal", "Rescaling Method"=enum."Single level", "Soft Threshold?"=TRUE}, "Wavelet Transform Type"=enum."Discrete"} ("Wavelet Analysis Options")) -> (Variant=w101:variant)
          }
          frame "Fluorescence Decay_Decay Pre-Processing:# Folds" {
            n68 = To Variant(anything=u32 1) -> (Variant=w103:variant)
          }
          frame "Fluorescence Decay_Decay Pre-Processing:1-Normalize Decay" {
            n69 = To Variant(anything=FALSE) -> (Variant=w105:variant)
          }
          frame "Fluorescence Decay_Decay Pre-Processing:[0-1]-Normalize Decay" {
            n70 = To Variant(anything=FALSE) -> (Variant=w107:variant)
          }
          frame "Fluorescence Decay_Decay Pre-Processing:Additional Points" {
            n71 = To Variant(anything=u32 100) -> (Variant=w109:variant)
          }
          frame "Fluorescence Decay_Decay Pre-Processing:Background Definition Range" {
            n72 = To Variant(anything=T17 {"Min Gate"=0.0, "Max Gate"=8e-10} ("Background Definition Range")) -> (Variant=w111:variant)
          }
          frame "Fluorescence Decay_Decay Pre-Processing:Background Subtraction" {
            n73 = To Variant(anything=FALSE) -> (Variant=w113:variant)
          }
          frame "Fluorescence Decay_Decay Pre-Processing:Baseline Subtraction Method" {
            n74 = To Variant(anything=AlliGator_Baseline_Subtraction_Method."Min" ("Baseline Subtraction Method")) -> (Variant=w115:variant)
          }
          frame "Fluorescence Decay_Decay Pre-Processing:Constant Background" {
            n75 = To Variant(anything=0.0) -> (Variant=w117:variant)
          }
          frame "Fluorescence Decay_Decay Pre-Processing:Decay Shift Parameters" {
            n76 = To Variant(anything=T19 {"Type"=enum."Default", "Shift"=0.0, "Threshold"=0.1, "Rotate"=FALSE} ("Decay Shift Parameters")) -> (Variant=w119:variant)
          }
          frame "Fluorescence Decay_Decay Pre-Processing:Extrapolate Decay" {
            n77 = To Variant(anything=FALSE) -> (Variant=w121:variant)
          }
          frame "Fluorescence Decay_Decay Pre-Processing:Fold Decay" {
            n78 = To Variant(anything=FALSE) -> (Variant=w123:variant)
          }
          frame "Fluorescence Decay_Decay Pre-Processing:Head Fraction" {
            n79 = To Variant(anything=0.5) -> (Variant=w125:variant)
          }
          frame "Fluorescence Decay_Decay Pre-Processing:Decay Pre-Processing Operations Order" {
            n80 = To Variant(anything=string[] ["Background subtraction", "Revert", "Smoothen", "Straighten", "Shift", "Extrapolate", "Normalize", "Fold"] ("Operation Order")) -> (Variant=w127:variant)
          }
          frame "Fluorescence Decay_Decay Pre-Processing:Pixel-Normalize Decay" {
            n81 = To Variant(anything=FALSE) -> (Variant=w129:variant)
          }
          frame "Fluorescence Decay_Decay Pre-Processing:Reverse Gates" {
            n82 = To Variant(anything=FALSE) -> (Variant=w131:variant)
          }
          frame "Fluorescence Decay_Decay Pre-Processing:Shift Decay" {
            n83 = To Variant(anything=FALSE) -> (Variant=w133:variant)
          }
          frame "Fluorescence Decay_Decay Pre-Processing:Smoothen Decay" {
            n84 = To Variant(anything=FALSE) -> (Variant=w135:variant)
          }
          frame "Fluorescence Decay_Decay Pre-Processing:Smoothing Parameter" {
            n85 = To Variant(anything=-1.0 ("Min Peak Value")) -> (Variant=w137:variant)
          }
          frame "Fluorescence Decay_Decay Pre-Processing:Straighten Decay" {
            n86 = To Variant(anything=FALSE) -> (Variant=w139:variant)
          }
          frame "Fluorescence Decay_Decay Pre-Processing:Tail Fraction" {
            n87 = To Variant(anything=0.5) -> (Variant=w141:variant)
          }
          frame "Fluorescence Decay_Decay Pre-Processing:Use Cursors" {
            n88 = To Variant(anything=FALSE) -> (Variant=w143:variant)
          }
          frame "Fluorescence Decay_Decay Pre-Processing:Use Decay Pre-Processing" {
            n89 = To Variant(anything=FALSE) -> (Variant=w145:variant)
          }
          frame "Fluorescence Decay_Decay Pre-Processing:Use Periodicity" {
            n90 = To Variant(anything=FALSE) -> (Variant=w147:variant)
          }
          frame "Fluorescence Decay_Decay Pre-Processing:Verbose Decay Pre-Processing" {
            n91 = To Variant(anything=TRUE) -> (Variant=w149:variant)
          }
          frame "Fluorescence Decay_Fit Options:Fit Options" {
            n92 = To Variant(anything=T21 {"Show Fit Residuals"=TRUE, "Fit Model"=enum."1-Exponential", "Residual Type"=enum."Standard", "Max Decay Percentile"=100.0, "Min Decay Percentile"=0.0, "Show Full Decay"=TRUE, "Weights"=enum."1/Variance", "Fitting Method"=enum."Least Square", "Compute Parameter Uncertainties"=TRUE, "Periodic Boundaries"=TRUE, "Model Calculation"=enum."Convolution", "Period"=1.2500000000000001e-08, "Termination Criteria"={"Max Iterations"=200, "Max Function Calls"=1000, "Max Time"=10.0, "Function Tolerance"=1e-06, "Parameter Tolerance"=1e-06, "Gradient Tolerance"=1e-06, "Min Lambda"=1e-06, "Max Lambda"=1000000.0, "Initial Tick Count"=0}, "Offset Resolution"=5e-11, "Use Local IRF"=FALSE, "Fitting Algorithm"=enum."Levenberg-Marquardt"} ("Fit Options")) -> (Variant=w151:variant)
          }
          frame "Fluorescence Decay_Fit Options:Use Data Information Laser Period" {
            n93 = To Variant(anything=TRUE) -> (Variant=w153:variant)
          }
          frame "Fluorescence Decay_Fit Options:Use Legacy Fitting Approach" {
            n94 = To Variant(anything=FALSE) -> (Variant=w155:variant)
          }
          frame "Fluorescence Decay_Fit Parameters:Displayed Fit Parameters" {
            w158 = T70[] [] items=["Offset", "Baseline", "A_1", "tau_1", "A_2", "tau_2", "<tau>_a", "f1_a", "f2_a", "<tau>_i", "f1_i", "f2_i", "-", "R^2", "Chi^2"] ("Array")
            n95 = To Variant(anything=w158) -> (Variant=w157:variant)
          }
          frame "Fluorescence Decay_Fit Parameters:Export Tabulated Results" {
            n96 = To Variant(anything=FALSE) -> (Variant=w159:variant)
          }
          frame "Fluorescence Decay_Fit Parameters:Fit Parameter Constraints" {
            n97 = To Variant(anything=T28[] [] ("Fit Parameter Constraints")) -> (Variant=w161:variant)
          }
          frame "Fluorescence Decay_Fit Parameters:Guess Parameter Names" {
            w164 = T29[] [] items=["Offset", "Baseline", "A_1", "tau_1", "A_2", "tau_2"] ("Guess Parameters Names")
            n98 = To Variant(anything=w164) -> (Variant=w163:variant)
          }
          frame "Fluorescence Decay_Fit Parameters:Guess Parameter Values" {
            n99 = To Variant(anything=dbl[] []) -> (Variant=w165:variant)
          }
          frame "Fluorescence Decay_Fit Parameters:Guess Parameters Options" {
            n100 = To Variant(anything=AlliGator_Guess_Parameters_Options."Numerically estimated" ("Guess Parameters Options")) -> (Variant=w167:variant)
          }
          frame "Fluorescence Decay_Fit Parameters:MLE Baseline Offset Type" {
            n101 = To Variant(anything=MLE_Baseline_Offset_Type."Absolute" ("MLE Baseline Offset Type")) -> (Variant=w169:variant)
          }
          frame "Fluorescence Decay_Fit Parameters:MLE Baseline Offset" {
            n102 = To Variant(anything=0.0 ("MLE Baseline Offset")) -> (Variant=w171:variant)
          }
          frame "Fluorescence Decay_Styles:Decay Graph Color Array" {
            n103 = To Variant(anything=u32[] [1985280, 16711680, 6618880] ("Decay Graph Color Array")) -> (Variant=w173:variant)
          }
          frame "Fluorescence Decay_Styles:Show Last Decay Only" {
            n104 = To Variant(anything=FALSE) -> (Variant=w175:variant)
          }
          frame "GUI:Last Run Version" {
            n105 = To Variant(anything="") -> (Variant=w177:variant)
          }
          frame "GUI:Visible Settings Tab", Default {
            n106 = To Variant(anything=0) -> (Variant=w179:variant)
          }
          frame "Lifetime Analysis:Decay Analysis Parameters" {
            n107 = To Variant(anything=T19 {"Type"=enum."Default", "Shift"=0.0, "Threshold"=0.0, "Rotate"=TRUE} ("IRF Analysis Method")) -> (Variant=w181:variant)
          }
          frame "Lifetime Analysis:Lifetime Map Active" {
            n108 = To Variant(anything=FALSE) -> (Variant=w183:variant)
          }
          frame "Miscellaneous:# Logical Processors Used" {
            n109 = CPU Information() -> (4:w188:i32)  [unwired: 3 out]
            n110 = Quotient & Remainder(x=w188, y=2) -> (floor(x/y)=w186:i32)  [unwired: 1 out]
            n111 = To Variant(anything=w186) -> (Variant=w185:variant)
          }
          frame "Miscellaneous:Beep after Script" {
            n112 = To Variant(anything=TRUE) -> (Variant=w189:variant)
          }
          frame "Miscellaneous:Beep on Error" {
            n113 = To Variant(anything=TRUE) -> (Variant=w191:variant)
          }
          frame "Miscellaneous:Exported Gate Image Settings" {
            n114 = To Variant(anything=T32 {"bitness"=TRUE, " Min Value"=-inf, " Max Value"=inf} ("Exported Gate Image Settings")) -> (Variant=w193:variant)
          }
          frame "Miscellaneous:Histogram Options" {
            n115 = To Variant(anything=T33 {"Bin Size"=nan, "Bin Number"=100, "Bin Option"=enum."Bin Number", "Min Value"=-inf, "Max Value"=inf, "Filter NaN & Infinite Values"=TRUE, "Frequency Plot"=FALSE, "Align Bins"=TRUE, "Bin Location"=enum."Left", "Project Outside Values"=FALSE, "Max Histogram Size"=100000} ("Histogram Options")) -> (Variant=w195:variant)
          }
          frame "Miscellaneous:Include Loading in Timing" {
            n116 = To Variant(anything=FALSE) -> (Variant=w197:variant)
          }
          frame "Miscellaneous:ROI Description Max Characters" {
            n117 = To Variant(anything=256) -> (Variant=w199:variant)
          }
          frame "Miscellaneous:Saved Image File Format" {
            n118 = To Variant(anything=Image_Save_File_Format."PNG" ("Saved Image File Format")) -> (Variant=w201:variant)
          }
          frame "Miscellaneous:Transparent Mask Color" {
            n119 = To Variant(anything=u32 16777216 ("Mask Color (Black)")) -> (Variant=w203:variant)
          }
          frame "Miscellaneous:Verbose Error Mode" {
            n120 = To Variant(anything=TRUE) -> (Variant=w205:variant)
          }
          frame "Miscellaneous:Verbose Mode" {
            n121 = To Variant(anything=FALSE) -> (Variant=w207:variant)
          }
          frame "Miscellaneous:Verbose Settings Mode" {
            n122 = To Variant(anything=FALSE) -> (Variant=w209:variant)
          }
          frame "Phasor Calibration:Backup Calibration Type" {
            n123 = To Variant(anything=T37."Nearest Valid Calibration" ("Backup Calibration")) -> (Variant=w211:variant)
          }
          frame "Phasor Calibration:Calibration Lifetime" {
            n124 = To Variant(anything=dbl[unit] 0.0 ("Calibration Lifetime")) -> (Variant=w213:variant)
          }
          frame "Phasor Calibration:Calibration Map Algorithm" {
            n125 = To Variant(anything=AlliGator_Calibration_Map_Algorithm."Min Distance" ("Calibration Map Algorithm")) -> (Variant=w215:variant)
          }
          frame "Phasor Calibration:Calibration Type" {
            n126 = To Variant(anything=Phasor_Calibration_Type."None" ("Calibration Type")) -> (Variant=w217:variant)
          }
          frame "Phasor Calibration:Use Backup Calibration if needed" {
            n127 = To Variant(anything=FALSE) -> (Variant=w219:variant)
          }
          frame "Phasor Graph:Define Shortest Lifetime as" {
            n128 = To Variant(anything=AlliGator_Phasor_Reference_Associated_with_Shortest_Lifetime."Reference 1" ("Define Shortest Lifetime as")) -> (Variant=w221:variant)
          }
          frame "Phasor Graph:Phasor Frequency" {
            w224 = dbl[unit] 80000000.0  # MHz
            n129 = To Variant(anything=w224) -> (Variant=w223:variant)
          }
          frame "Phasor Graph:Phasor Graph Active" {
            n130 = To Variant(anything=TRUE) -> (Variant=w225:variant)
          }
          frame "Phasor Graph:Phasor Ratio Type" {
            n131 = To Variant(anything=Phasor_Ratio_Type."Amplitude-weighted" ("Phasor Ratio Type")) -> (Variant=w227:variant)
          }
          frame "Phasor Graph:Phasor SDV Options" {
            n132 = To Variant(anything=T42 {"Compute Estimated SDV"=FALSE, "# Replicas"=1000, "Use Estimated Average Phasor"=FALSE} ("Phasor SDV Options")) -> (Variant=w229:variant)
          }
          frame "Phasor Graph:Pixel-level Phasor Computation" {
            n133 = To Variant(anything=FALSE) -> (Variant=w231:variant)
          }
          frame "Phasor Graph:Save Phasor Graph" {
            n134 = To Variant(anything=FALSE) -> (Variant=w233:variant)
          }
          frame "Phasor Plot:All Image ROIs" {
            n135 = To Variant(anything=FALSE) -> (Variant=w235:variant)
          }
          frame "Phasor Plot:All Phasor Plot ROIs" {
            n136 = To Variant(anything=FALSE) -> (Variant=w237:variant)
          }
          frame "Phasor Plot:Blend Overlay with Phasor Background" {
            n137 = To Variant(anything=FALSE) -> (Variant=w239:variant)
          }
          frame "Phasor Plot:Cumulative Phasor Plot" {
            n138 = To Variant(anything=FALSE) -> (Variant=w241:variant)
          }
          frame "Phasor Plot:Draw Reference Segment" {
            n139 = To Variant(anything=TRUE) -> (Variant=w243:variant)
          }
          frame "Phasor Plot:Exponential Fading" {
            n140 = To Variant(anything=FALSE) -> (Variant=w245:variant)
          }
          frame "Phasor Plot:Phasor Plot Active" {
            n141 = To Variant(anything=TRUE) -> (Variant=w247:variant)
          }
          frame "Phasor Plot:Phasor Plot Graphics Options" {
            n142 = To Variant(anything=T43 {"UC Color"=0, "Show UC Tau Ticks"=FALSE, "SEPL Color"=7171459, "Show SEPL Tau Ticks"=FALSE, "Axes Color"=0, "Show (g,s) Ticks"=TRUE, "Show UC"=TRUE, "Show SEPL"=FALSE, "Show Axes"=TRUE, "Show UC Tau Labels"=FALSE, "Show SEPL Tau Labels"=FALSE, "Show (g,s) Labels"=TRUE, "UC Label Size"=16, "UC Label Distance"=2.0, "SEPL Label Size"=16, "SEPL Label Distance"=1.5, "Axes Label Size"=18, "Axes Label Distance"=3.0} ("Phasor Plot Graphics Options")) -> (Variant=w249:variant)
          }
          frame "Phasor Plot:Phasor Plot Size" {
            n143 = To Variant(anything=T44 {"H"=512, "V"=512, "Margin"=0.5} ("Phasor Plot Size")) -> (Variant=w251:variant)
          }
          frame "Phasor Plot:Phasor Plot Smoothing Options" {
            n144 = To Variant(anything=T45 {"Use Phasor Plot Smoothing"=FALSE, "Kernel Type"=enum."Uniform", "Bin"=1, "Algorithm"=enum."Rapid"} ("Phasor Plot Smoothing Options")) -> (Variant=w253:variant)
          }
          frame "Phasor Plot:Phasor Ratio Color Map Type" {
            n145 = To Variant(anything=T48."Interpolate Reference Colors" ("Phasor Ratio Color Map Type")) -> (Variant=w255:variant)
          }
          frame "Phasor Plot:Phasor Ratio Color Map" {
            n146 = To Variant(anything="Rainbow") -> (Variant=w257:variant)
          }
          frame "Phasor Plot:Phasor Ratio Color-Coded Quantity" {
            n147 = To Variant(anything=AlliGator_Phasor_Ratio_Color-Coded_Quantity."Phasor Ratio (f1 or a1)" ("Displayed Quantity")) -> (Variant=w259:variant)
          }
          frame "Phasor Plot:Phasor Ratio Decay Range" {
            n148 = To Variant(anything=0.1 ("Phasor Ratio Decay Range")) -> (Variant=w261:variant)
          }
          frame "Phasor Plot:Phasor Ratio Display Range" {
            n149 = To Variant(anything=cluster{"Min":dbl, "Max":dbl} {"Min"=0.0, "Max"=1.0} ("Phasor Ratio Display Range")) -> (Variant=w263:variant)
          }
          frame "Phasor Plot:Phasor Ratio Reference Colors" {
            n150 = To Variant(anything=T50 {"Reference 1"=6618880, "Reference 2"=16711680, "Boundary"=9868950} ("Phasor Ratio Reference Colors")) -> (Variant=w265:variant)
          }
          frame "Phasor Plot:Reference Radius" {
            n151 = To Variant(anything=3 ("Reference Radius")) -> (Variant=w267:variant)
          }
          frame "Phasor Plot:Save Phasor Plot" {
            n152 = To Variant(anything=FALSE) -> (Variant=w269:variant)
          }
          frame "Phasor Plot:Selected Image ROI(s)" {
            n153 = To Variant(anything=FALSE) -> (Variant=w271:variant)
          }
          frame "Phasor Plot:Selected Phasor Plot ROI(s)" {
            n154 = To Variant(anything=FALSE) -> (Variant=w273:variant)
          }
          frame "Phasor Plot:Show Color Map Vertices" {
            n155 = To Variant(anything=FALSE) -> (Variant=w275:variant)
          }
          frame "Phasor Plot:Show References" {
            n156 = To Variant(anything=FALSE) -> (Variant=w277:variant)
          }
          frame "Phasor Plot:Store Phasor Harmonics" {
            n157 = To Variant(anything=FALSE) -> (Variant=w279:variant)
          }
          frame "Phasor Plot:Use Phasor Brightness" {
            n158 = To Variant(anything=FALSE) -> (Variant=w281:variant)
          }
          frame "Phasor Plot:User-Defined Quantity" {
            n159 = To Variant(anything="") -> (Variant=w283:variant)
          }
          frame "Plugins:Python Settings" {
            n160 = To Variant(anything=T51 {"Python Version"="3.9", "Use PATH definition"=TRUE, "Python.exe Path"=path "", "Include Example Plugins"=TRUE} ("Python Settings")) -> (Variant=w285:variant)
          }
          frame "Single-Exponential Phasor Locus (SEPL):Decay & IRF Parameters" {
            n161 = To Variant(anything=T52 {"Lifetime"=1.0, "IRF Offset"=0.0, "IRF Period"=1.2500000000000001e-08, "Normalized Decays"=FALSE, "IRF Model"=enum."Dirac", "IRF Parameter 1"=0.1} ("Phasor Explorer Decay & IRF Parameters")) -> (Variant=w287:variant)
          }
          frame "Single-Exponential Phasor Locus (SEPL):Display Parameters" {
            n162 = To Variant(anything=T54 {"# Points"=1000, "Ramp Type"=enum."Logarithmic", "Type of Series"=enum."1-Exp Decays", "Min tau"=1.0000000000000002e-12, "Max tau"=1.0000000000000001e-07, "Include 0"=TRUE, "Include Infinity"=TRUE} ("SEPL Display Parameters")) -> (Variant=w289:variant)
          }
          frame "Single-Exponential Phasor Locus (SEPL):Gate Parameters" {
            n163 = To Variant(anything=T56 {"First Gate Start"=0.0, "Use Gate Center"=FALSE, "Gate Width"=0.0, "Gate Step"=0.0, "# Gates"=inf, "Gate Type"=enum."Square", "Edge Width"=0.0, "Top Slope"=0.0, "Reversed Sawtooth?"=FALSE, "Analytical Computation"=FALSE, "Integration"=enum."Item 0", "Tolerance"=0.001, "# Steps"=1000.0, "Type of User-defined Function"=enum."IRF", "Use Gate Step"=FALSE} ("Phasor Explorer Gate Parameters")) -> (Variant=w291:variant)
          }
          frame "Single-Exponential Phasor Locus (SEPL):Phasor Parameters" {
            n164 = To Variant(anything=T59 {"Harmonic Frequency"=80000000.0, "Use f* = 1/D Frequency"=FALSE, "Calibrated Phasor"=TRUE, "Calibration Lifetime"=0.0, "Phasor Calculation"=enum."Analytical Formula", "SEPL Type"=enum."UC", "# Gates"=1000.0, "Square Gate Width"=0.0, "Show Ticks"=FALSE} ("SEPL Calibration Parameters")) -> (Variant=w293:variant)
          }
          frame "Single-Exponential Phasor Locus (SEPL):User-defined Gate" {
            n165 = To Variant(anything=T62 {"X Array"=[], "Y Array"=[]} ("Plot")) -> (Variant=w295:variant)
          }
          frame "Single-Exponential Phasor Locus (SEPL):User-defined IRF" {
            n166 = To Variant(anything=T62 {"X Array"=[], "Y Array"=[]} ("Plot")) -> (Variant=w297:variant)
          }
          frame "Source Image:Auto-Adjust Contrast" {
            n167 = To Variant(anything=FALSE) -> (Variant=w299:variant)
          }
          frame "Source Image:Blend Overlay with Image Background" {
            n168 = To Variant(anything=FALSE) -> (Variant=w301:variant)
          }
          frame "Source Image:High Count Pixels Rejection Options" {
            n169 = To Variant(anything=T63 {"Background High Threshold Factor"=inf, "Fixed High Background Threshold"=inf, "Reject High Count Pixels"=FALSE, "High Percentile"=0.0} ("High Count Pixels Rejection Options")) -> (Variant=w303:variant)
          }
          frame "Source Image:Histogram Lower Percentile" {
            n170 = To Variant(anything=1.0) -> (Variant=w305:variant)
          }
          frame "Source Image:Histogram Upper Percentile" {
            n171 = To Variant(anything=1.0) -> (Variant=w307:variant)
          }
          frame "Source Image:Hot Pixel Removal" {
            n172 = To Variant(anything=T64 {"Remove Screamers"=FALSE, "Delta"=inf, "Equalize Histogram"=FALSE, "Percentile"=0.0, "Hot Pixel Mask Image"=path "", "Use Hot Pixel Mask"=FALSE} ("Image Display Options")) -> (Variant=w309:variant)
          }
          frame "Source Image:Image Binning Options" {
            n173 = To Variant(anything=T65 {"Use Image Binning"=FALSE, "X Bin"=1, "Y Bin"=1} ("Image Binning Options")) -> (Variant=w311:variant)
          }
          frame "Source Image:Image Histogram Active" {
            n174 = To Variant(anything=TRUE) -> (Variant=w313:variant)
          }
          frame "Source Image:Image Smoothing Options" {
            n175 = To Variant(anything=T66 {"Use Image Smoothing"=FALSE, "Kernel Type"=enum."Uniform", "Bin"=1, "Algorithm"=enum."Rapid"} ("Image Binning Options")) -> (Variant=w315:variant)
          }
          frame "Source Image:Intensity Threshold" {
            n176 = To Variant(anything=500.0) -> (Variant=w317:variant)
          }
          frame "Source Image:Invert Binary Mask" {
            n177 = To Variant(anything=FALSE) -> (Variant=w319:variant)
          }
          frame "Source Image:Low Count Pixels Rejection Options" {
            n178 = To Variant(anything=T67 {"Background Low Threshold Factor"=0.0, "Fixed Low Background Threshold"=0.0, "Reject Low Count Pixels"=FALSE, "Low Percentile"=0.0} ("Low Count Pixels Rejection Options")) -> (Variant=w321:variant)
          }
          frame "Source Image:Overlay Analyzed ROI Center" {
            n179 = To Variant(anything=FALSE) -> (Variant=w323:variant)
          }
          frame "Source Image:Peak Threshold" {
            n180 = To Variant(anything=500.0) -> (Variant=w325:variant)
          }
          frame "Source Image:ROI Center Color" {
            n181 = To Variant(anything=u32 16711680) -> (Variant=w327:variant)
          }
          frame "Source Image:ROI Diameter" {
            n182 = To Variant(anything=12) -> (Variant=w329:variant)
          }
          frame "Source Image:Save Source Image" {
            n183 = To Variant(anything=FALSE) -> (Variant=w331:variant)
          }
          frame "Source Image:Use Fixed ROI Diameter" {
            n184 = To Variant(anything=FALSE) -> (Variant=w333:variant)
          }
          frame "Source Image:Use Image Brightness" {
            n185 = To Variant(anything=FALSE) -> (Variant=w335:variant)
          }
          frame "Source Image:Use Image Histogram for Contrast" {
            n186 = To Variant(anything=TRUE) -> (Variant=w337:variant)
          }
          frame "Source Image:Scale Bar Options" {
            n187 = To Variant(anything=T68 {"Show Scale Bar Overlay"=FALSE, "Scale Bar Length"=9.999999999999999e-06, "Scale Bar Color"=0, "Scale Bar X"=20, "Scale Bar Y"=20, "Scale Bar Height"=1e-06} ("Scale Bar Options")) -> (Variant=w339:variant)
          }
          frame "Source Image:Image Resolution (Pixel Size)" {
            w342 = dbl[unit] 1e-07  # Image Resolution (Pixel Size)
            n188 = To Variant(anything=w342) -> (Variant=w341:variant)
          }
          frame "Source Image:Flatfield Correction" {
            n189 = To Variant(anything=T69 {"Flatfield Estimation Options"={"Sampling Grid Size X"=256, "Sampling Grid Size Y"=256, "Polynomial Degree"=5}, "Background Options"={"Estimate Background"=TRUE, "Background Estimation Size"=32, "Niblack Deviation Factor [0. 1]"=0.2}, "Correction Factor"=1.1} ("Flatfield Correction")) -> (Variant=w343:variant)
          }
          frame "Source Image:Show Dead Left Columns Correction" {
            n190 = To Variant(anything=FALSE) -> (Variant=w346:variant)
          }
          frame "Source Image:Image Pre-Processing Operations Order" {
            n191 = To Variant(anything=FALSE) -> (Variant=w348:variant)
          }
          frame "Source Image:Dead Left Columns Correction" {
            n192 = To Variant(anything=FALSE) -> (Variant=w350:variant)
          }
          frame "Source Image:Overlay ROI Median" {
            n193 = To Variant(anything=FALSE) -> (Variant=w352:variant)
          }
          frame "Source Image:Median Overlay Color" {
            n194 = To Variant(anything=u32 6618880) -> (Variant=w354:variant)
          }
          frame "Time Traces:Intensity Correction File" {
            n195 = To Variant(anything=path "") -> (Variant=w355:variant)
          }
          frame "Time Traces:Time Step" {
            n196 = To Variant(anything=dbl[unit] 1.0 ("Time Step")) -> (Variant=w357:variant)
          }
          frame "Time Traces:Use File Timestamp" {
            n197 = To Variant(anything=TRUE) -> (Variant=w359:variant)
          }
          frame "Time Traces:Use Intensity Correction File" {
            n198 = To Variant(anything=FALSE) -> (Variant=w361:variant)
          }
        }
        n199 = call "AlliGator Settings Storage.vi"("Get(F)/Set"=TRUE, "AlliGator Settings List"=w26, "Error In"=w27, "Variant Data in"=w29) -> ("Error Out"=w30:errorcluster)  [unwired: 6 in, 1 out]
      }
    }
  }
  n200 = call "AlliGator Settings Event Refnum.vi"("AlliGator Settings Event"=w3, "Error In"=w1) -> ("Error Out"=→"error out":errorcluster)  [unwired: 6 in, 1 out]
